vi "9759 Properties.vi"() -> ()   [LabVIEW 2015, in "NI 9759 RevB Custom Device.lvlib"]
uses:
  NI 9759 RevB Custom Device.lvlib
panel:
  in  "Tab Control":enum32{"Main", "System"}(tab)
  in  "Main.ControlCal":string="Main.ControlCal"
  in  "Main.PositionCal":string="Main.PositionCal"
  in  "Main.FPGA Resource":string="Main.FPGA Resource"
  in  "Main.IP Address":string="Main.IP Address"
  in  "Main.FPGA Location":string="Main.FPGA Location"
  in  "Main.DCMCreated":string="Main.DCMCreated"
  in  "Main.Cam Captures":string="Main.Cam Captures"
  in  "Main.CompiledData":string="Main.CompiledData"
  in  "Main.CPU":string="Main.CPU"
  in  "Main.validBitfile":string="Main.validBitfile"
  in  "IP.bitfile name":string="IP.bitfile name"
  in  "Main.bitfile EPS version":string="Main.bitfile EPS version"
  in  "Main.Bitfile":string="Main.Bitfile"
  in  "Main.Device Address":string="Main.Device Address"
  in  "System.Settings":string="System.Settings"
  in  "System.State Indexes":string="System.State Indexes"
  in  "System.Status":string="System.Status"
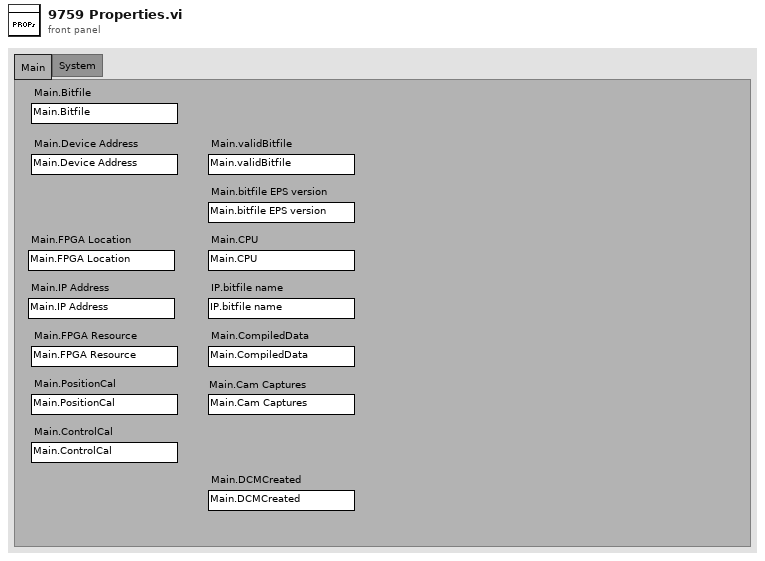
[diagram p1: front panel]
diagram:
